vi "Read Aux.vi"(11 "JoystickDevRef":T1={"Device"=enum."USB 1"}) -> ()   [LabVIEW 2018]
uses:
  <vilib>/Rock Robotics/WPI/Joystick/WPI_JoystickDevRef.ctl
  <vilib>/Rock Robotics/WPI/Joystick/WPI_JoystickDeviceEnum.ctl
  Robot Global Data.vi
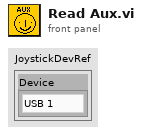
[diagram p1: front panel]
types:
  T1 = typedef "WPI_JoystickDevRef.ctl" = cluster{"Device":T2}
  T2 = typedef "WPI_JoystickDeviceEnum.ctl" = enum16{"USB 0", "USB 1", "USB 2", "USB 3", "USB 4", "USB 5"}
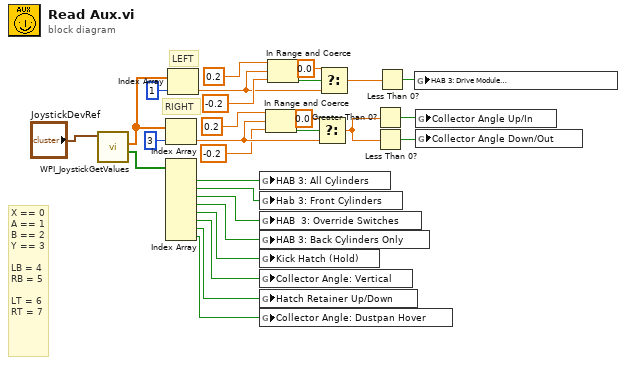
[diagram p0: block diagram]
diagram:
  # "LEFT"
  # "RIGHT"
  # "X == 0\nA == 1\nB == 2\nY == 3\n\nLB = 4\nRB = 5\n\nLT = 6\nRT = 7"
  n1 = call <vilib>:"WPI_JoystickGetValues.vi"("JoystickDevRef"="JoystickDevRef") -> ("Buttons"=w28:bool[], "Axes"=w10:dbl[])  [unwired: 6 in, 3 out]
  n2 = Index Array(array=w10, index=3) -> (element=w17:dbl)
  n3 = Index Array(array=w28) -> (element #1=w26:bool, element #2=w25:bool, element #3=w24:bool, element #4=w23:bool, element #5=w22:bool, element #6=w21:bool, element #7=w20:bool, element #8=w19:bool)  [unwired: 8 in]
  n4 = Index Array(array=w10, index=1) -> (element=w2:dbl)
  n5 = global write "Robot Global Data.vi" "HAB 3: All Cylinders"(w26) -> ()
  n6 = global write "Robot Global Data.vi" "Hab 3: Front Cylinders"(w25) -> ()
  n7 = global write "Robot Global Data.vi" "HAB  3: Override Switches"(w24) -> ()
  n8 = global write "Robot Global Data.vi" "HAB 3: Back Cylinders Only"(w23) -> ()
  n9 = global write "Robot Global Data.vi" "Kick Hatch (Hold)"(w22) -> ()
  n10 = global write "Robot Global Data.vi" "Collector Angle: Vertical"(w21) -> ()
  n11 = global write "Robot Global Data.vi" "Hatch Retainer Up/Down"(w20) -> ()
  n12 = global write "Robot Global Data.vi" "Collector Angle: Dustpan Hover"(w19) -> ()
  n13 = In Range and Coerce(upper limit=0.2, x=w17, lower limit=-0.2) -> (In Range?=w18:bool)  [unwired: 1 out]
  n14 = In Range and Coerce(upper limit=0.2, x=w2, lower limit=-0.2) -> (In Range?=w8:bool)  [unwired: 1 out]
  n15 = Select(t=0.0, s=w18, f=w17) -> (s? t:f=w13:dbl)
  n16 = Select(t=0.0, s=w8, f=w2) -> (s? t:f=w4:dbl)
  n17 = Greater Than 0?(x=w13) -> (x > 0?=w12:bool)
  n18 = Less Than 0?(x=w13) -> (x < 0?=w11:bool)
  n19 = Less Than 0?(x=w4) -> (x < 0?=w3:bool)
  n20 = global write "Robot Global Data.vi" "HAB 3: Drive Module\n(FORWARD)"(w3) -> ()
  n21 = global write "Robot Global Data.vi" "Collector Angle Up/In"(w12) -> ()
  n22 = global write "Robot Global Data.vi" "Collector Angle Down/Out"(w11) -> ()
